vi "Global-Initialize.vi"(8 "error in (no error)":errorcluster, 10 "active error checking":bool=TRUE, 11 "VISA resource name":refnum<visa-resource-name>) -> (0 "error out":errorcluster, 3 "VISA resource name out":refnum<visa-resource-name>)   [LabVIEW 2016, in "Agilent 415X Series.lvlib"]
doc: "This VI queries the HP 4155A/56A for presence of extra source/monitor units including the two SMUs, the GNDU, and the PGU housed in the expansion box."
uses:
  Agilent 415X Series.lvlib
  Private/Global.vi
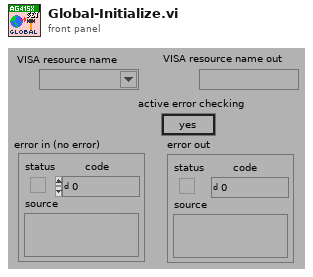
[diagram p1: front panel]
types:
  T1 = cluster{bool, bool, bool, bool, bool, bool, "active error checking":bool, "VISA resource name":refnum<visa-resource-name>}
  T2 = cluster{"valid instrument":bool, "GNDU present":bool, "SMU5 present":bool, "SMU6 present":bool, "PGU1 present":bool, "PGU2 present":bool, "active error checking":bool, "instr. handler":refnum<visa-resource-name>}[]
  T3 = cluster{"valid instrument":bool, "GNDU present":bool, "SMU5 present":bool, "SMU6 present":bool, "PGU1 present":bool, "PGU2 present":bool, "active error checking":bool, "VISA resource name":refnum<visa-resource-name>}[]
  T4 = cluster{bool, bool, bool, bool, bool, bool, "active error checking":bool, "VISA resource name":refnum<visa-resource-name>}[]
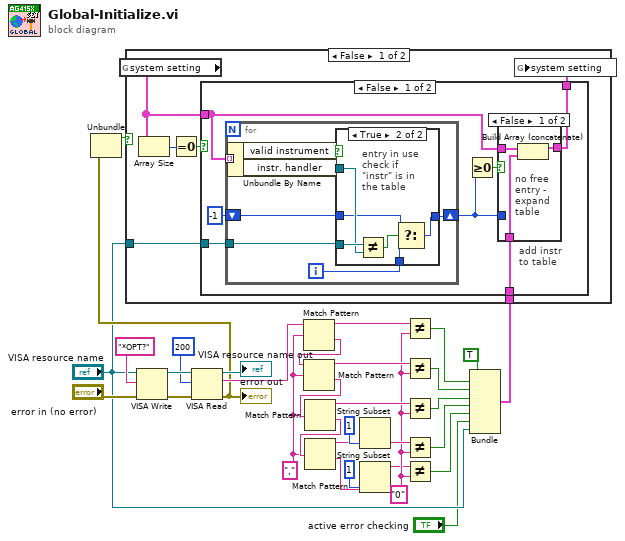
[diagram p0: block diagram]
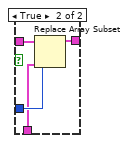
[diagram p2: hidden frame]
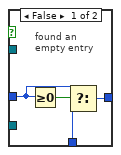
[diagram p3: hidden frame]
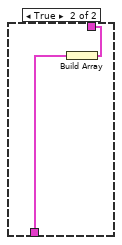
[diagram p4: hidden frame]
diagram:
  w4 = "0"
  w6 = ","
  n1 = VISA Write(VISA resource name="VISA resource name", write buffer="*OPT?", error in (no error)="error in (no error)") -> (VISA resource name out=w31:refnum<visa-resource-name>, error out=w32:errorcluster)  [unwired: 1 out]
  n2 = VISA Read(VISA resource name=w31, byte count=200, error in (no error)=w32) -> (VISA resource name out=→"VISA resource name out":refnum<visa-resource-name>, read buffer=w26:string, error out=w20:errorcluster)  [unwired: 1 out]
  "error out" <- w20
  n3 = Unbundle(w20) -> ("status"=w21:bool)  [unwired: 2 out]
  n4 = Match Pattern(string=w26, regular expression=w6) -> (before substring=w18:string, after substring=w28:string)  [unwired: 1 in, 2 out]
  n5 = Match Pattern(string=w28, regular expression=w6) -> (before substring=w17:string, after substring=w27:string)  [unwired: 1 in, 2 out]
  n6 = Match Pattern(string=w27, regular expression=w6) -> (before substring=w16:string, after substring=w7:string)  [unwired: 1 in, 2 out]
  n7 = Match Pattern(string=w7, regular expression=w6) -> (before substring=w5:string, after substring=w8:string)  [unwired: 1 in, 2 out]
  n8 = String Subset(string=w5, length (rest)=1) -> (substring=w15:string)  [unwired: 1 in]
  n9 = String Subset(string=w8, length (rest)=1) -> (substring=w3:string)  [unwired: 1 in]
  n10 = Not Equal?(x=w18, y=w4) -> (x != y?=w14:bool)
  n11 = Not Equal?(x=w17, y=w4) -> (x != y?=w13:bool)
  n12 = Not Equal?(x=w16, y=w4) -> (x != y?=w12:bool)
  n13 = Not Equal?(x=w15, y=w4) -> (x != y?=w11:bool)
  n14 = Not Equal?(x=w3, y=w4) -> (x != y?=w2:bool)
  n15 = Bundle(TRUE, w14, w13, w12, w11, w2, "active error checking"="active error checking", "VISA resource name"="VISA resource name") -> (w22:T1)  [unwired: 1 in]
  n16 = case shown="False" w21 {
    tunnel: w22 -> [w35 _]
    tunnel: "VISA resource name" -> [w34 _]
    frame False {
      n17 = global read "Global.vi" "system setting"() -> (w33:T2)
      n18 = Array Size(array=w33) -> (size(s)=w38:i32)
      n19 = Equal To 0?(x=w38) -> (x = 0?=w37:bool)
      n20 = case shown="False" w37 {
        tunnel: w35 -> [w41 w70]
        tunnel: w33 -> [w40 _]
        tunnel: w34 -> [w44 _]
        tunnel: [w39 w71] -> w36
        frame False {
          # "add instr\nto table"
          n21 = for {
            shift-right: [w58] -> w42
            shift-left: -1 ("empty-entry-index") -> [w59]
            tunnel: w44 -> [w53]
            tunnel: w40 -> [w55] mode=indexing
            i -> [w56]
            n22 = Unbundle By Name(w55) -> ("valid instrument"=w54:bool, "instr. handler"=w57:refnum<visa-resource-name>)
            n23 = case shown="True" w54 {
              tunnel: w59 -> [w61 w65]
              tunnel: [w63 w64] -> w58
              tunnel: w53 -> [_ w69]
              tunnel: w57 -> [_ w68]
              tunnel: w56 -> [w60 w66]
              frame False {
                # "found an\nempty entry"
                n24 = Greater Or Equal To 0?(x=w61) -> (x >= 0?=w62:bool)
                n25 = Select(t=w61, s=w62, f=w60) -> (s? t:f=w63:i32)
              }
              frame True {
                # "entry in use\ncheck if\n\"instr\" is in\nthe table"
                n26 = Not Equal?(x=w69, y=w68) -> (x != y?=w67:bool)
                n27 = Select(t=w65, s=w67, f=w66) -> (s? t:f=w64:i32)
              }
            }
          }
          n28 = Greater Or Equal To 0?(x=w42) -> (x >= 0?=w43:bool)
          n29 = case shown="False" w43 {
            tunnel: w42 -> [_ w52]
            tunnel: w41 -> [w46 w49]
            tunnel: w40 -> [w48 w51]
            tunnel: [w47 w50] -> w39
            frame False {
              # "no free\nentry -\nexpand\ntable"
              n30 = Build Array (concatenate)(w48, w46) -> (w47:T3)
            }
            frame True {
              n31 = Replace Array Subset(array=w51, new element=w49, index=w52) -> (w50:T2)
            }
          }
        }
        frame True {
          n32 = Build Array(w70) -> (w71:T4)
        }
      }
      n33 = global write "Global.vi" "system setting"(w36) -> ()
    }
    frame True {
      # "a previous error exists"
    }
  }
